vi "ArrayToSprdSht.vi"(4 "Column End":i32, 6 "Row End":i32, 9 "TextArray":string[][](array[string]), 10 "report file path":path, 11 "template (empty)":path) -> ()   [LabVIEW 2017]
uses:
  <vilib>/addons/_office/_exclsub.llb/font.ctl
  <vilib>/Utility/NIReport.llb/Append Text Table to Report (wrap).vi
  <vilib>/Utility/NIReport.llb/NI_report.lvclass
  <vilib>/Utility/NIReport.llb/Excel/NI_Excel.lvclass
  <vilib>/addons/_office/NI_ReportGenerationToolkit.lvlib
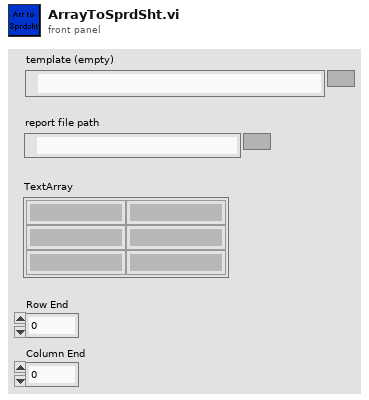
[diagram p1: front panel]
types:
  T1 = cluster{"on/off":bool, "weight":i32, "color":u32}
  T2 = typedef "NI_ReportGenerationToolkit.lvlib/font.ctl" = cluster{"font name":string, "font size":dbl, "bold":u16, "italic":u16, "underline":u16, "strike through":u16, "font color":u32}
  T3 = enum16{"Standard Report", "HTML", "Word", "Excel"}
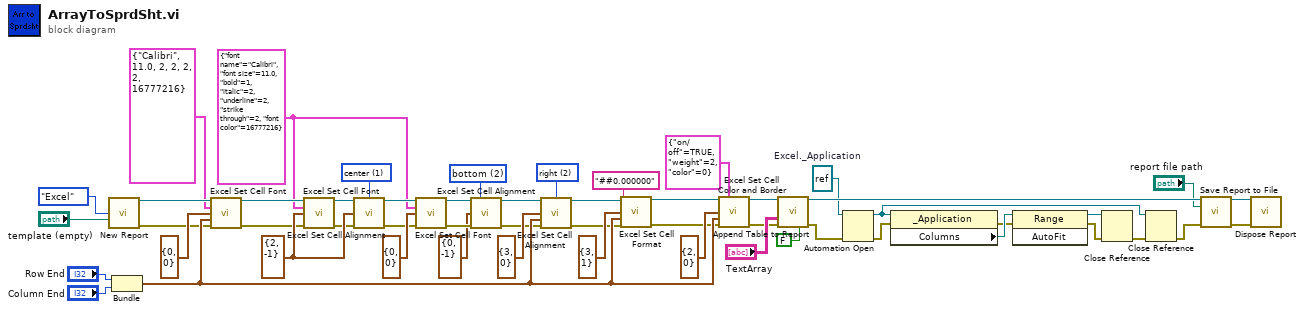
[diagram p0: block diagram]
diagram:
  w3 = 2 items=["top", "center", "bottom"] ("vertical alignment (top)")
  w25 = refnum<k7> refnum  # Excel._Application
  w39 = T2 {"font name"="Calibri", "font size"=11.0, "bold"=1, "italic"=2, "underline"=2, "strike through"=2, "font color"=16777216} ("font")
  w51 = 2 items=["left", "center", "right"] ("horizontal alignment (left)")
  w42 = cluster{"row":i32, "column":i32} {"row"=2, "column"=-1} ("start (-1, -1)")
  w52 = 1 items=["left", "center", "right"] ("horizontal alignment (left)")
  n1 = call <vilib>:"New Report.vi"("report type"=T3."Excel", "template (empty)"="template (empty)") -> ("report out"=w46:refnum<class "NI_report.lvclass">, "error out"=w15:errorcluster)  [unwired: 12 in]
  n2 = Bundle("Row End"="Row End", "Column End"="Column End") -> (w27:cluster{"Row End":i32, "Column End":i32})  [unwired: 1 in]
  n3 = call <vilib>:"Excel Set Cell Font.vi"("report in"=w46, "font"=T2 {"font name"="Calibri", "font size"=11.0, "bold"=2, "italic"=2, "underline"=2, "strike through"=2, "font color"=16777216}, "start (-1, -1)"=cluster{"row":i32, "column":i32} {"row"=0, "column"=0}, "end (-1, -1)"=w27, "error in (no error)"=w15) -> ("report out"=w43:refnum<class "NI_report.lvclass">, "error out"=w14:errorcluster)  [unwired: 9 in]
  n4 = call <vilib>:"Excel Set Cell Font.vi"("report in"=w43, "font"=w39, "start (-1, -1)"=w42, "error in (no error)"=w14) -> ("report out"=w41:refnum<class "NI_report.lvclass">, "error out"=w13:errorcluster)  [unwired: 10 in]
  n5 = call <vilib>:"Excel Set Cell Alignment.vi"("report in"=w41, "horizontal alignment (left)"=w52, "start (-1, -1)"=w42, "error in (no error)"=w13) -> ("report out"=w40:refnum<class "NI_report.lvclass">, "error out"=w12:errorcluster)  [unwired: 10 in]
  n6 = call <vilib>:"Excel Set Cell Font.vi"("report in"=w40, "font"=w39, "start (-1, -1)"=cluster{"row":i32, "column":i32} {"row"=0, "column"=0}, "error in (no error)"=w12) -> ("report out"=w8:refnum<class "NI_report.lvclass">, "error out"=w7:errorcluster)  [unwired: 10 in]
  n7 = call <vilib>:"Excel Set Cell Alignment.vi"("report in"=w8, "vertical alignment (top)"=w3, "start (-1, -1)"=cluster{"row":i32, "column":i32} {"row"=0, "column"=-1}, "error in (no error)"=w7) -> ("report out"=w5:refnum<class "NI_report.lvclass">, "error out"=w6:errorcluster)  [unwired: 10 in]
  n8 = call <vilib>:"Excel Set Cell Alignment.vi"("report in"=w5, "horizontal alignment (left)"=w51, "start (-1, -1)"=cluster{"row":i32, "column":i32} {"row"=3, "column"=0}, "end (-1, -1)"=w27, "error in (no error)"=w6) -> ("report out"=w48:refnum<class "NI_report.lvclass">, "error out"=w11:errorcluster)  [unwired: 9 in]
  n9 = call <vilib>:"Excel Set Cell Format.vi"("report in"=w48, "number format"="##0.000000", "start (-1, -1)"=cluster{"row":i32, "column":i32} {"row"=3, "column"=1}, "end (-1, -1)"=w27, "error in (no error)"=w11) -> ("report out"=w32:refnum<class "NI_report.lvclass">, "error out"=w10:errorcluster)  [unwired: 9 in]
  n10 = call <vilib>:"Excel Set Cell Color and Border.vi"("report in"=w32, "inside border"=T1 {"on/off"=TRUE, "weight"=2, "color"=0}, "start (-1, -1)"=cluster{"row":i32, "column":i32} {"row"=2, "column"=0}, "end (-1, -1)"=w27, "error in (no error)"=w10) -> ("report out"=w26:refnum<class "NI_report.lvclass">, "error out"=w9:errorcluster)  [unwired: 9 in]
  n11 = call-poly <vilib>:"Append Table to Report.vi"("report in"=w26, "text data"="TextArray", "error in (no error)"=w9, "show grid lines (YES)"=FALSE) -> ("report out"=w35:refnum<class "NI_report.lvclass">, "error out"=w17:errorcluster)  [unwired: 8 in, 2 out]
  n12 = Automation Open(error in (no error)=w17, Automation Refnum=w25) -> (Automation Refnum=w18:refnum<k7>, error out=w24:errorcluster)  [unwired: 2 in]
  n13 = property class="_Application"(reference=w18, error in=w24) -> (error out=w22:errorcluster, "Columns"=w23:refnum<k7>)  [unwired: 1 out]
  n14 = invoke class="Range" method="AutoFit"(reference=w23, error in=w22) -> (reference out=w21:refnum<k7>, error out=w20:errorcluster)  [unwired: 1 in, 1 out]
  n15 = Close Reference(reference=w21, error in (no error)=w20) -> (error out=w19:errorcluster)
  n16 = Close Reference(reference=w18, error in (no error)=w19) -> (error out=w16:errorcluster)
  n17 = call-dynamic "Save Report to File.vi"("report in"=w35, "report file path"="report file path", "error in (no error)"=w16) -> ("report out"=w2:refnum<class "NI_report.lvclass">, "error out"=w1:errorcluster)  [unwired: 11 in]
  n18 = call-dynamic "Dispose Report.vi"("report in"=w2, "error in (no error)"=w1) -> ()  [unwired: 13 in, 1 out]
